vi "Freeze_Check.vi"(8 "error in (no error)":errorcluster, 11 "DataCluster in":T2={"Core"={"Current VI Reference"=refnum, "Close Panel on Exit?"=FALSE, "Exit"=FALSE, "Initialized?"=FALSE}, "Connections"={"cDAQ"={"Task"="ThermTask", "Connected"=FALSE, "Active"=FALSE, "ID"=""}, "Camera"={"Session"="", "Connected"=FALSE, "Active"=FALSE, "Placeholder"=refnum}, "PSU"={"Port"="", "Connected"=FALSE, "Active"=FALSE}, "Arduino"={"Port"="", "Connected"=FALSE, "Active"=FALSE}}, "Data Acquisition"={"Setup"={"Label"="_41", "Operator"="", "Notes"="", "TempGrad"=1.0, "TargetTemp"=-20.0, "Sample Volume"=1.0}, "Camera"={"Image"=refnum, "Save Image"=refnum, "Image Frequency"=20, "Rectangle"={"Left"=0, "Top"=0, "Right"=0, "Bottom"=0, "Rotation"=0.0}, "Calibration"={"Top Left"={"X"=0.0, "Y"=0.0}, "Top Right"={"X"=0.0, "Y"=0.0}, "Bottom Left"={"X"=0.0, "Y"=0.0}, "Bottom Right"={"X"=0.0, "Y"=0.0}, "Fixpoint"={"X"=0.0, "Y"=0.0}, "Scan Area"=0.0, "Fixpoint Area"=0.0, "Well Pixels"=[], "Valid"=FALSE}, "FocusPos"=0, "Display Mapping"=10}, "Thermistor"={"Sample Size"=5, "Calibration"={"B0.100"=[3450.0, 3450.0, 3450.0, 3450.0, 3450.0, 3450.0, 3450.0, 3450.0], "R25"=[10.74, 10.74, 10.74, 10.74, 10.74, 10.74, 10.74, 10.74], "c"=[], "State"=[], "V_S"=10.0, "R_S"=10.0}, "Timing Mode"=14713}, "Partition"={"Data"=[], "Cell Label"="", "Cell Color"=0, "Height"=10, "Width"=16, "Grid"=[]}, "Queue"={"Size"=5, "Queue"=refnum}, "Sample Rate"=240, "Active"=FALSE, "Ready"=FALSE, "Graph Mode"=0, "Gradient Buffer"=2}, "Control"={"Sample Rate"=20, "PID gains"={"proportional gain (Kc)"=1.0, "integral time (Ti, min)"=0.01, "derivative time (Td, min)"=0.0}}, "Manual Temp Control"={"TargetTemp"=1.0, "Mode"=0, "Active"=FALSE}} {"Manual Temp Control"."Mode" items=["Cool", "Heat"]; "Manual Temp Control"."TargetTemp" min=-40.0 max=40.0 step=0.5 format="%#_g °C"; "Control"."PID gains"."derivative time (Td, min)" format="%.3f"; "Control"."PID gains"."integral time (Ti, min)" format="%.3f"; "Control"."PID gains"."proportional gain (Kc)" format="%.3f"; "Control"."Sample Rate" min=1 max=20 step=1 format="%.0f Samples/sec"; "Data Acquisition"."Gradient Buffer" min=2 max=30 step=1; "Data Acquisition"."Graph Mode" items=["Thermistor Temperature", "Camera Temperature"]; "Data Acquisition"."Thermistor"."Timing Mode" items=["Automatic"=16097, "High Resolution"=10195, "High Speed"=14712, "Best 50 Hz Rejection"=14713, "Best 60 Hz Rejection"=14714, "Custom"=10137]; "Data Acquisition"."Thermistor"."Calibration"."R_S" min=0.1 max=1000.0 format="%#_g kOhm"; "Data Acquisition"."Thermistor"."Calibration"."V_S" min=5.0 max=48.0 format="%#_g V"; "Data Acquisition"."Thermistor"."Calibration"."R25" min=0.1 max=1000.0 format="%#_g kOhm"; "Data Acquisition"."Thermistor"."Calibration"."B0.100" min=100.0 max=10000.0 format="%#_g K"; "Data Acquisition"."Thermistor"."Sample Size" min=1 max=200; "Data Acquisition"."Sample Rate" min=20 max=240 format="%.0f samples/min"; "Data Acquisition"."Queue"."Size" min=1 max=200; "Data Acquisition"."Camera"."Display Mapping" items=["Default"=10, "Most Significant Bits"=11, "Full Dynamic"=12, "Downshift"=13, "Given Range"=14, "90% Dynamic"=15, "Given Percent Range"=16]; "Data Acquisition"."Camera"."Calibration"."Fixpoint"."Y" format="%.2f"; "Data Acquisition"."Camera"."Calibration"."Fixpoint"."X" format="%.2f"; "Data Acquisition"."Camera"."Calibration"."Top Left"."Y" format="%.2f"; "Data Acquisition"."Camera"."Calibration"."Top Left"."X" format="%.2f"; "Data Acquisition"."Camera"."Calibration"."Top Right"."Y" format="%.2f"; "Data Acquisition"."Camera"."Calibration"."Top Right"."X" format="%.2f"; "Data Acquisition"."Camera"."Calibration"."Bottom Left"."Y" format="%.2f"; "Data Acquisition"."Camera"."Calibration"."Bottom Left"."X" format="%.2f"; "Data Acquisition"."Camera"."Calibration"."Bottom Right"."Y" format="%.2f"; "Data Acquisition"."Camera"."Calibration"."Bottom Right"."X" format="%.2f"; "Data Acquisition"."Camera"."Rectangle"."Rotation" min=-90.0 max=90.0 step=1.0 format="%.2f"; "Data Acquisition"."Camera"."Rectangle"."Left" scale=0.0..1024.0; "Data Acquisition"."Camera"."Rectangle"."Right" scale=0.0..1024.0; "Data Acquisition"."Camera"."Image Frequency" min=1 max=60 step=1; "Data Acquisition"."Setup"."Sample Volume" min=0.0 max=500.0 format="%#_g µL"; "Data Acquisition"."Setup"."TargetTemp" min=-40.0 max=40.0 step=0.5 format="%#_g °C"; "Data Acquisition"."Setup"."TempGrad" min=-100.0 max=100.0 step=0.1 format="%#_g °C/min"}) -> (0 "error out":errorcluster)   [LabVIEW 2020]
uses:
  DataCluster.ctl
  <vilib>/userDefined/High Color/IMAQdx.ctl
  <vilib>/vision/Image Controls.llb/IMAQ Image.ctl
panel:
  out "Proc_Img":T1(plugin-control)
  in  "Threshold":i32=15 min=0 max=255
  in  "RGB/Binary":enum32{"RGB", "Binary"}(radio)
  out "Cal_Img":T1(plugin-control)
  in  "Image":i32(slide) caption="Horizontal Slider" min=-2 max=94 scale=0.0..94.0
  in  "Path":path
  # "Calibration Image"
  # "Processing Image"
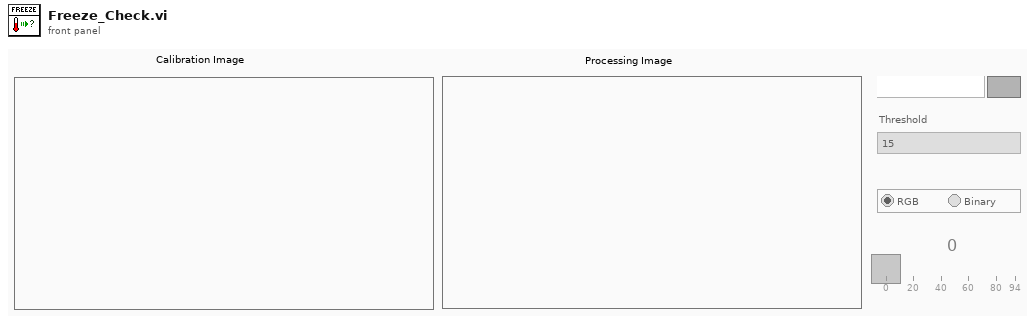
[diagram p1: front panel]
types:
  T1 = typedef "IMAQ Image.ctl" = refnum<image>
  T2 = typedef "DataCluster.ctl" = cluster{"Core":cluster{"Current VI Reference":refnum<vi>, "Close Panel on Exit?":bool, "Exit":bool, "Initialized?":bool}, "Connections":cluster{"cDAQ":cluster{"Task":refnum<k21>, "Connected":bool, "Active":bool, "ID":string}, "Camera":cluster{"Session":T3, "Connected":bool, "Active":bool, "Placeholder":T1}, "PSU":cluster{"Port":refnum<visa-resource-name>, "Connected":bool, "Active":bool}, "Arduino":cluster{"Port":refnum<visa-resource-name>, "Connected":bool, "Active":bool}}, "Data Acquisition":cluster{"Setup":cluster{"Label":string, "Operator":string, "Notes":string, "TempGrad":dbl, "TargetTemp":dbl, "Sample Volume":dbl}, "Camera":cluster{"Image":T1, "Save Image":T1, "Image Frequency":i32, "Rectangle":T4, "Calibration":cluster{"Top Left":T5, "Top Right":T5, "Bottom Left":T5, "Bottom Right":T5, "Fixpoint":T5, "Scan Area":dbl, "Fixpoint Area":dbl, "Well Pixels":cluster{"X":i32, "Y":i32}[][], "Valid":bool}, "FocusPos":u32, "Display Mapping":u32}, "Thermistor":cluster{"Sample Size":i32, "Calibration":cluster{"B0.100":dbl[], "R25":dbl[], "c":dbl[][], "State":bool[], "V_S":dbl, "R_S":dbl}, "Timing Mode":i32}, "Partition":cluster{"Data":string[][], "Cell Label":string, "Cell Color":u32, "Height":i32, "Width":i32, "Grid":string[][]}, "Queue":cluster{"Size":i32, "Queue":refnum<queue>}, "Sample Rate":i32, "Active":bool, "Ready":bool, "Graph Mode":u16, "Gradient Buffer":i32}, "Control":cluster{"Sample Rate":i32, "PID gains":cluster{"proportional gain (Kc)":dbl, "integral time (Ti, min)":dbl, "derivative time (Td, min)":dbl}}, "Manual Temp Control":cluster{"TargetTemp":dbl, "Mode":u16, "Active":bool}}
  T3 = typedef "IMAQdx.ctl" = refnum<k21>
  T4 = typedef "IMAQ Rectangle" = cluster{"Left":i32, "Top":i32, "Right":i32, "Bottom":i32, "Rotation":dbl}
  T5 = typedef "IMAQ Point" = cluster{"X":sgl, "Y":sgl}
  T6 = enum8{"Enabled", "Disabled", "Disabled and Grayed Out"}
  T7 = typedef "Image Type" = u32
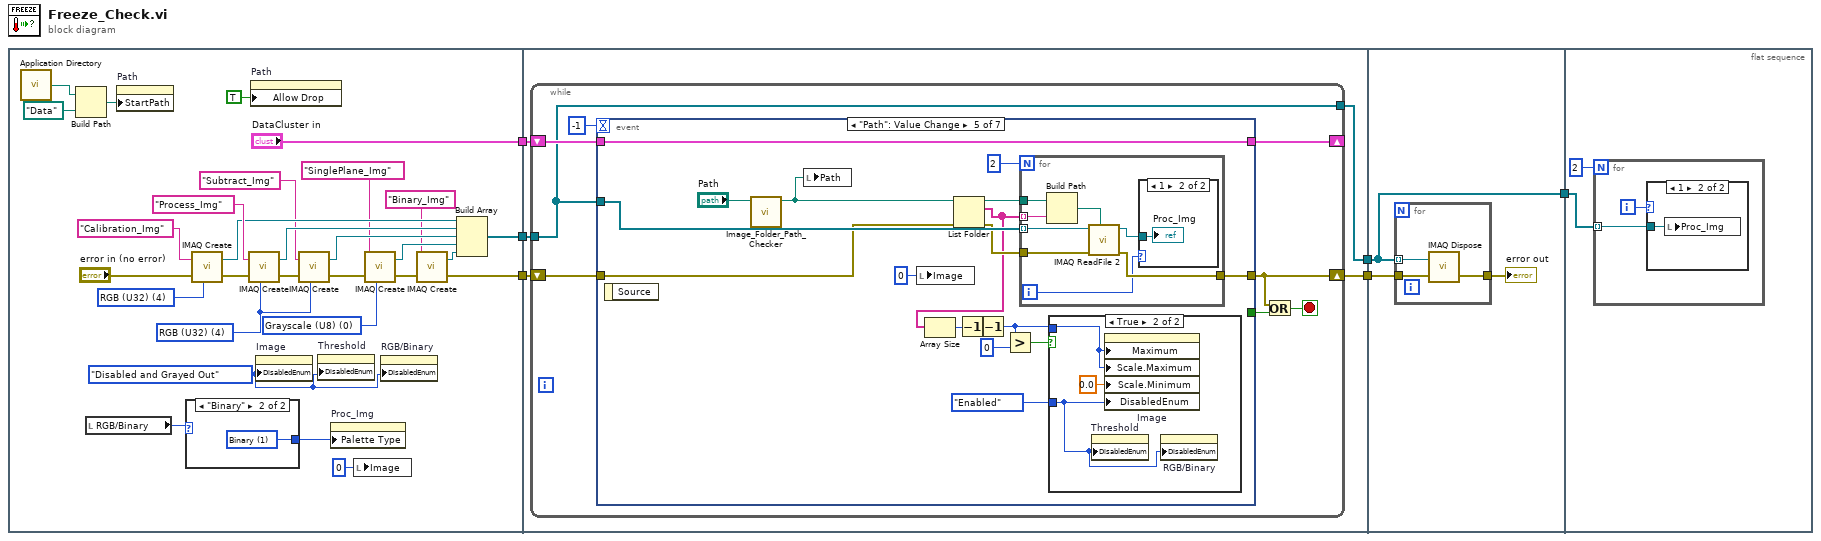
[diagram p0: block diagram]
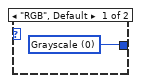
[diagram p2: hidden frame]
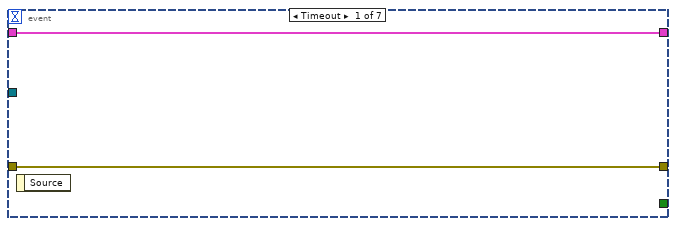
[diagram p3: hidden frame]
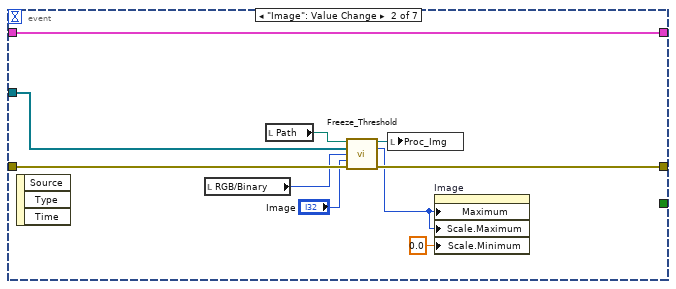
[diagram p4: hidden frame]
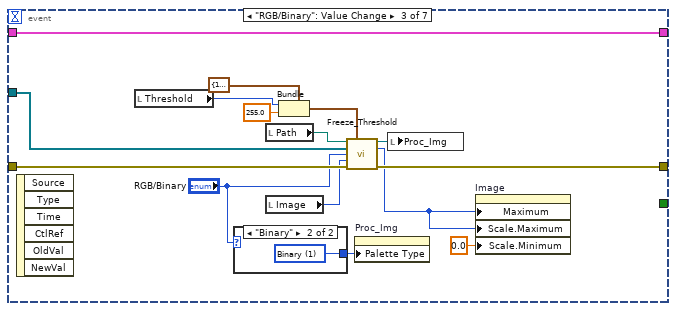
[diagram p5: hidden frame]
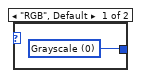
[diagram p6: hidden frame]
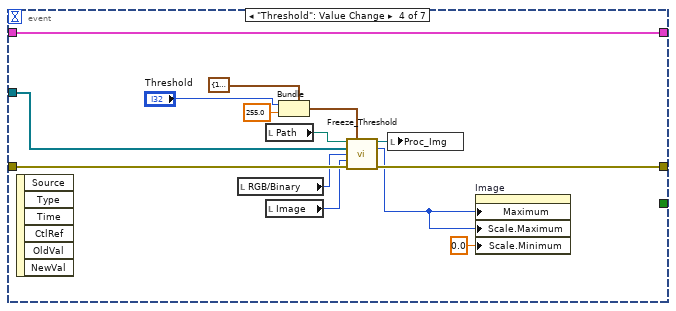
[diagram p7: hidden frame]
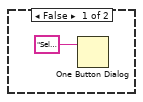
[diagram p8: hidden frame]
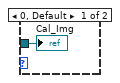
[diagram p9: hidden frame]
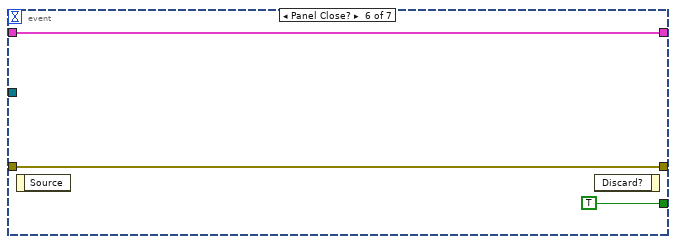
[diagram p10: hidden frame]
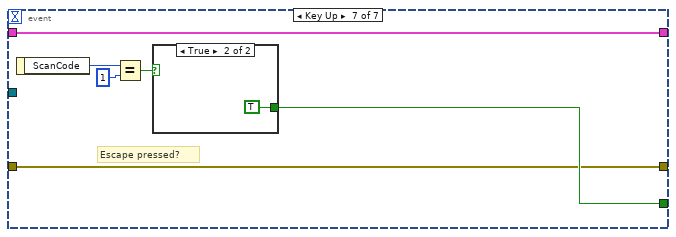
[diagram p11: hidden frame]
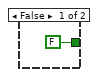
[diagram p12: hidden frame]
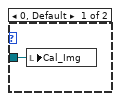
[diagram p13: hidden frame]
diagram:
  n1 = flat-sequence {
    tunnel: [w16] -> w6
    tunnel: ["DataCluster in"] -> w5
    tunnel: [w26] -> w4
    tunnel: w6 -> [w42]
    tunnel: w5 -> [w41]
    tunnel: w4 -> [w39]
    tunnel: [w40] -> w3
    tunnel: [w38] -> w2
    tunnel: w3 -> [w137]
    tunnel: w2 -> [w136]
    tunnel: [w136] -> w1
    tunnel: w1 -> [w142]
    frame #0 {
      w12 = T7 0 items=["Grayscale (U8)", "Grayscale (I16)", "Grayscale (SGL)", "Complex (CSG)", "RGB (U32)", "HSL (U32)", "RGB (U64)", "Grayscale (U16)"] ("Image Type")
      w10 = T6."Disabled and Grayed Out" ("Disabled")
      w13 = T7 4 items=["Grayscale (U8)", "Grayscale (I16)", "Grayscale (SGL)", "Complex (CSG)", "RGB (U32)", "HSL (U32)", "RGB (U64)", "Grayscale (U16)"] ("Image Type")
      w35 = T7 4 items=["Grayscale (U8)", "Grayscale (I16)", "Grayscale (SGL)", "Complex (CSG)", "RGB (U32)", "HSL (U32)", "RGB (U64)", "Grayscale (U16)"] ("Image Type")
      n2 = call <vilib>:"Application Directory.vi"() -> ("Application Directory"=w29:path)
      n3 = Build Path(base path=w29, name or relative path=path "Data") -> (appended path=w28:path)
      n4 = local read "RGB/Binary"() -> (w11:enum32{"RGB", "Binary"})
      n5 = property on="Path" class="Path"("StartPath"=w28) -> ()  [unwired: 2 in, 2 out]
      n6 = case shown="\"Binary\"" w11 {
        tunnel: [w36 w37] -> w8
        frame "RGB", Default {
          w36 = u32 0 items=["Grayscale", "Binary", "Gradient", "Rainbow", "Temperature", "User Defined", "Binary 16 Bit", "Gradient 16 Bit", "Rainbow 16 Bit", "Temperature 16 Bit", "User Defined 16 Bit"] ("Palette:Palette Type")
        }
        frame "Binary" {
          w37 = u32 1 items=["Grayscale", "Binary", "Gradient", "Rainbow", "Temperature", "User Defined", "Binary 16 Bit", "Gradient 16 Bit", "Rainbow 16 Bit", "Temperature 16 Bit", "User Defined 16 Bit"] ("Palette:Palette Type")
        }
      }
      n7 = call "IMAQ Create"("Image Name"="Calibration_Img", "Image Type"=w35, "error in (no error)"="error in (no error)") -> ("New Image"=w25:T1, "error out"=w32:errorcluster)  [unwired: 2 in]
      n8 = call "IMAQ Create"("Image Name"="Process_Img", "Image Type"=w13, "error in (no error)"=w32) -> ("New Image"=w24:T1, "error out"=w22:errorcluster)  [unwired: 2 in]
      n9 = property on="Path" class="Path"("Allow Drop"=TRUE ("Allow Dropping")) -> ()  [unwired: 2 in, 2 out]
      n10 = property on="Image" class="Slide (strict)"("DisabledEnum"=w10) -> ()  [unwired: 2 in, 2 out]
      n11 = call "IMAQ Create"("Image Name"="Subtract_Img", "Image Type"=w13, "error in (no error)"=w22) -> ("New Image"=w21:T1, "error out"=w20:errorcluster)  [unwired: 2 in]
      n12 = property on="Threshold" class="DigNum (strict)"("DisabledEnum"=w10) -> ()  [unwired: 2 in, 2 out]
      n13 = property on="Proc_Img" class="ImageControl"("Palette Type"=w8) -> ()  [unwired: 2 in, 2 out]
      n14 = local write "Image"(0 ("Image")) -> ()
      n15 = call "IMAQ Create"("Image Name"="SinglePlane_Img", "Image Type"=w12, "error in (no error)"=w20) -> ("New Image"=w18:T1, "error out"=w17:errorcluster)  [unwired: 2 in]
      n16 = property on="RGB/Binary" class="RadioBtnsControl (strict)"("DisabledEnum"=w10) -> ()  [unwired: 2 in, 2 out]
      n17 = call "IMAQ Create"("Image Name"="Binary_Img", "error in (no error)"=w17) -> ("New Image"=w14:T1, "error out"=w16:errorcluster)  [unwired: 3 in]
      n18 = Build Array(w25, w24, w21, w18, w14) -> (w26:T1[])
    }
    frame #1 {
      n19 = while {
        shift-right: [w50] -> _
        shift-left: w41 -> [w49]
        shift-right: [w44] -> w40
        shift-left: w42 -> [w45]
        tunnel: w39 -> [w43]
        tunnel: [w43] -> w38
        stop <- w46 stop-if-true
        n20 = event shown="[4] \"Path\": Value Change" {
          selector: _ -> [_ _ _ _ _ _ _]
          dyn-events: _ -> [_ _ _ _ _ _ _]
          timeout: -1 -> [_ _ _ _ _ _ _]
          tunnel: w49 -> [w51 w62 w77 w93 w110 w125 w128]
          tunnel: [w51 w62 w77 w93 w110 w125 w128] -> w50
          tunnel: [_ _ _ _ _ TRUE w133] -> w48
          tunnel: [w52 w57 w73 w89 w102 w126 w129] -> w44
          tunnel: w45 -> [w52 w60 w75 w91 w104 w126 w129]
          tunnel: w43 -> [_ w58 w74 w90 w105 _ _]
          event Timeout {
            n21 = event-data() -> ()  [unwired: 1 in, 1 out]
          }
          event "Image": Value Change {
            n22 = event-data() -> ()  [unwired: 1 in, 3 out]
            n23 = local read "RGB/Binary"() -> (w55:enum32{"RGB", "Binary"})
            n24 = local read "Path"() -> (w61:path)
            n25 = call "Freeze_Threshold.vi"("Path"=w61, "Array"=w58, "RGB/Binary"=w55, "Image"="Image", "error in (no error)"=w60) -> ("Image out"=w56:T1, "Numeric"=w54:i32, "error out"=w57:errorcluster)  [unwired: 8 in]
            n26 = local write "Proc_Img"(w56) -> ()
            n27 = property on="Image" class="Slide (strict)"("Maximum"=w54, "Scale.Maximum"=w54, "Scale.Minimum"=0.0 ("Scale.Range:Minimum")) -> ()  [unwired: 2 in, 2 out]
          }
          event "RGB/Binary": Value Change {
            n28 = event-data() -> ()  [unwired: 1 in, 6 out]
            n29 = local read "Threshold"() -> (w66:i32)
            n30 = case shown="\"Binary\"" "RGB/Binary" {
              tunnel: [w78 w79] -> w63
              frame "RGB", Default {
                w78 = u32 0 items=["Grayscale", "Binary", "Gradient", "Rainbow", "Temperature", "User Defined", "Binary 16 Bit", "Gradient 16 Bit", "Rainbow 16 Bit", "Temperature 16 Bit", "User Defined 16 Bit"] ("Palette:Palette Type")
              }
              frame "Binary" {
                w79 = u32 1 items=["Grayscale", "Binary", "Gradient", "Rainbow", "Temperature", "User Defined", "Binary 16 Bit", "Gradient 16 Bit", "Rainbow 16 Bit", "Temperature 16 Bit", "User Defined 16 Bit"] ("Palette:Palette Type")
              }
            }
            n31 = local read "Path"() -> (w76:path)
            n32 = local read "Image"() -> (w71:i32)
            n33 = Bundle(cluster=cluster{"Lower value":sgl, "Upper value":sgl} {"Lower value"=128.0, "Upper value"=255.0} ("Range"), "Lower value"=w66, "Upper value"=sgl 255.0) -> (w65:cluster{"Lower value":sgl, "Upper value":sgl})
            n34 = call "Freeze_Threshold.vi"("Path"=w76, "Range"=w65, "Array"=w74, "RGB/Binary"="RGB/Binary", "Image"=w71, "error in (no error)"=w75) -> ("Image out"=w72:T1, "Numeric"=w69:i32, "error out"=w73:errorcluster)  [unwired: 7 in]
            n35 = property on="Proc_Img" class="ImageControl"("Palette Type"=w63) -> ()  [unwired: 2 in, 2 out]
            n36 = local write "Proc_Img"(w72) -> ()
            n37 = property on="Image" class="Slide (strict)"("Maximum"=w69, "Scale.Maximum"=w69, "Scale.Minimum"=0.0 ("Scale.Range:Minimum")) -> ()  [unwired: 2 in, 2 out]
          }
          event "Threshold": Value Change {
            n38 = event-data() -> ()  [unwired: 1 in, 6 out]
            n39 = local read "RGB/Binary"() -> (w81:enum32{"RGB", "Binary"})
            n40 = local read "Path"() -> (w92:path)
            n41 = local read "Image"() -> (w87:i32)
            n42 = Bundle(cluster=cluster{"Lower value":sgl, "Upper value":sgl} {"Lower value"=128.0, "Upper value"=255.0} ("Range"), "Lower value"="Threshold", "Upper value"=sgl 255.0) -> (w82:cluster{"Lower value":sgl, "Upper value":sgl})
            n43 = call "Freeze_Threshold.vi"("Path"=w92, "Range"=w82, "Array"=w90, "RGB/Binary"=w81, "Image"=w87, "error in (no error)"=w91) -> ("Image out"=w88:T1, "Numeric"=w85:i32, "error out"=w89:errorcluster)  [unwired: 7 in]
            n44 = local write "Proc_Img"(w88) -> ()
            n45 = property on="Image" class="Slide (strict)"("Maximum"=w85, "Scale.Maximum"=w85, "Scale.Minimum"=0.0 ("Scale.Range:Minimum")) -> ()  [unwired: 2 in, 2 out]
          }
          event "Path": Value Change {
            n46 = event-data() -> ()  [unwired: 1 in, 1 out]
            n47 = call "Image_Folder_Path_Checker.vi"("Path"="Path") -> ("appended path"=w108:path)  [unwired: 10 in]
            n48 = local write "Path"(w108) -> ()
            n49 = local write "Image"(0 ("Image")) -> ()
            n50 = List Folder(path=w108, error in=w104) -> (path out=w106:path, filenames=w101:string[], error out=w103:errorcluster)  [unwired: 2 in, 1 out]
            n51 = Array Size(array=w101) -> (size(s)=w100:i32)
            n52 = Decrement(x=w100) -> (x-1=w99:i32)
            n53 = Decrement(x=w99) -> (x-1=w96:i32)
            n54 = Greater?(x=w96, y=0) -> (0:w94:bool)
            n55 = for {
              N: 2 -> [_]
              tunnel: w106 -> [w122]
              tunnel: w101 -> [w121] mode=indexing
              tunnel: w105 -> [w119] mode=indexing
              tunnel: w103 -> [w118]
              tunnel: [w117] -> w102
              i -> [w116]
              n56 = Build Path(base path=w122, name or relative path=w121) -> (appended path=w120:path)
              n57 = call "IMAQ ReadFile 2"("File Path"=w120, "error in (no error)"=w118, "Image"=w119) -> ("error out"=w117:errorcluster, "Image Out"=w115:T1)  [unwired: 4 in, 3 out]
              n58 = case shown="1" w116 {
                tunnel: w115 -> [w123 w124]
                frame 0, Default {
                  "Cal_Img" <- w123
                }
                frame 1 {
                  "Proc_Img" <- w124
                }
              }
            }
            n59 = case shown="True" w94 {
              tunnel: T6."Enabled" ("Disabled") -> [_ w112]
              tunnel: w96 -> [_ w113]
              frame False {
                n60 = One Button Dialog(message="Selected folder contains no images.") -> ()  [unwired: 1 in, 1 out]
              }
              frame True {
                n61 = property on="Threshold" class="DigNum (strict)"("DisabledEnum"=w112) -> ()  [unwired: 2 in, 2 out]
                n62 = property on="Image" class="Slide (strict)"("Maximum"=w113, "Scale.Maximum"=w113, "Scale.Minimum"=0.0 ("Scale.Range:Minimum"), "DisabledEnum"=w112) -> ()  [unwired: 2 in, 2 out]
                n63 = property on="RGB/Binary" class="RadioBtnsControl (strict)"("DisabledEnum"=w112) -> ()  [unwired: 2 in, 2 out]
              }
            }
          }
          event Panel Close? {
            n64 = event-data() -> ()  [unwired: 1 in, 1 out]
            n65 = event-data() -> ()  [unwired: 2 in, 1 out]
          }
          event Key Up {
            # "Escape pressed?"
            n66 = event-data() -> ("ScanCode"=w132:i16)  [unwired: 1 in]
            n67 = Equal?(x=w132, y=i16 1) -> (x = y?=w130:bool)
            n68 = case shown="True" w130 {
              tunnel: [FALSE TRUE] -> w133
              frame False {
              }
              frame True {
              }
            }
          }
        }
        n69 = Or(x=w44, y=w48) -> (x .or. y?=w46:bool)
      }
    }
    frame #2 {
      n70 = for {
        tunnel: [w141] -> w138
        tunnel: w137 -> [w140]
        tunnel: w136 -> [w139] mode=indexing
        n71 = call "IMAQ Dispose"("Image"=w139, "error in (no error)"=w140) -> ("error out"=w141:errorcluster)  [unwired: 4 in]
      }
      "error out" <- w138
    }
    frame #3 {
      n72 = for {
        N: 2 -> [_]
        tunnel: w142 -> [w145] mode=indexing
        i -> [w144]
        n73 = case shown="1" w144 {
          tunnel: w145 -> [w146 w147]
          frame 0, Default {
            n74 = local write "Cal_Img"(w146) -> ()
          }
          frame 1 {
            n75 = local write "Proc_Img"(w147) -> ()
          }
        }
      }
    }
  }
